vi "Method.vi"(4 "Value":refnum<class "Abs_U16 Integer.lvclass">) -> (1 "Result":refnum<class "Abs_U16 Integer.lvclass">)   [LabVIEW 2021, in "Increment_U16.lvclass"]
uses:
  Increment_U16.lvclass
  Abs_Types/U16 Integer/Abs_U16 Integer.lvclass
  C:/Users/Tim/Documents/LabVIEW/2021/Data Classes/Source/Functions/Support/One Terminal/U16/AbsFunc_One Term_U16.lvclass
  C:/Users/Tim/Documents/LabVIEW/2021/Data Classes/Source/Abs_Types/U16 Integer/Abs_U16 Integer.lvclass
  Support/One Terminal/U16/AbsFunc_One Term_U16.lvclass/AbsFunc_One Term_U16.ctl
  Support/One Terminal/U16/Properties/Write Numeric A.vi
  Increment_U16.lvclass/Increment_U16.ctl
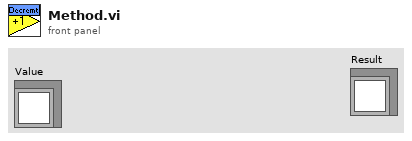
[diagram p1: front panel]
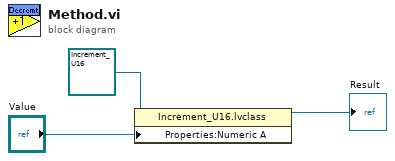
[diagram p0: block diagram]
diagram:
  n1 = property class="Increment_U16.lvclass"(reference=refnum<class "Increment_U16.lvclass"> refnum ("Decrement_DBL.lvclass"), "Properties:Numeric A"="Value") -> (reference out=→"Result":refnum<class "Increment_U16.lvclass">)  [unwired: 1 in, 1 out]
